vi "ValueChanged Callback.vi"(4 "onValueChanged":refnum<user-event>, 5 "Event Data":cluster{"sender":refnum<k24>, "e":refnum<k24>}, 6 "Control Ref":refnum<k24>, 7 "Event Common Data":T1) -> ()   [LabVIEW 2024, in "SourceGrid.lvlib" / "Custom Events.lvclass"]
uses:
  Custom Events.lvclass
  D:/git/Sourcegrid-LabVIEW/dll/SourceGrid.dll
  dll/SourceGrid.dll
  Cells/Cell Context/Cell Context.lvclass
  Custom Events.lvclass/Custom Events.ctl
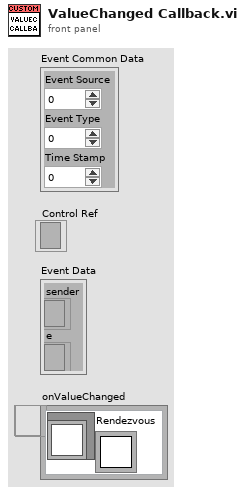
[diagram p1: front panel]
types:
  T1 = cluster{"Event Source":i32, "Event Type":u32, "Time Stamp":u32}
  T2 = typedef "Rendezvous RefNum" = refnum<k1>
  T3 = cluster{"Cell Context":refnum<class "Cell Context.lvclass">, "Rendezvous":T2}
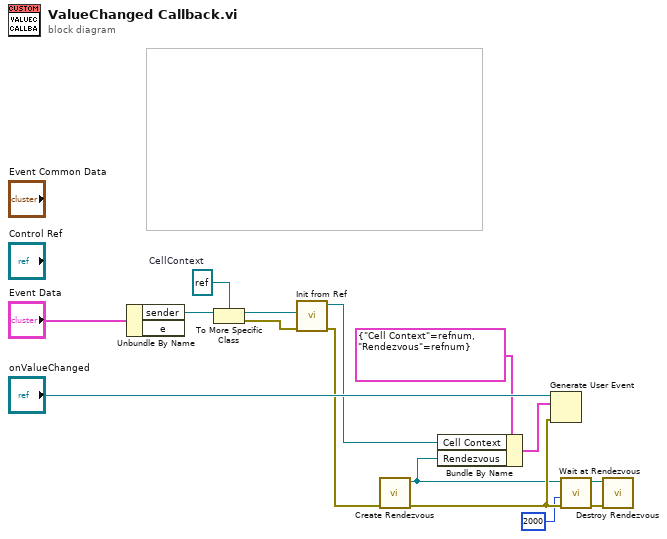
[diagram p0: block diagram]
diagram:
  w14 = refnum<k24> refnum  # CellContext
  n1 = Unbundle By Name("Event Data") -> ("sender"=w15:refnum<k24>)  [unwired: 1 out]
  n2 = To More Specific Class(target class=w14, reference=w15) -> (specific class reference=w10:refnum<k24>, error out=w13:errorcluster)  [unwired: 1 in]
  n3 = call "Init from Ref.vi"("error in"=w13, "CellContext .NET"=w10) -> ("error out"=w6:errorcluster, "Cell Context out"=w8:refnum<class "Cell Context.lvclass">)  [unwired: 8 in]
  n4 = call <vilib>:"Create Rendezvous.vi"("error in (no error)"=w6) -> ("error out"=w5:errorcluster, "rendezvous"=w1:T2)  [unwired: 4 in, 1 out]
  n5 = Bundle By Name(cluster=T3 {"Cell Context"=refnum, "Rendezvous"=refnum} ("onClick 2"), "Cell Context"=w8, "Rendezvous"=w1) -> (w7:T3)
  n6 = Generate User Event(user event="onValueChanged", event data cluster=w7, error in=w5) -> ()  [unwired: 1 in, 2 out]
  n7 = call <vilib>:"Wait at Rendezvous.vi"("error in (no error)"=w5, "ms timeout (-1)"=2000, "rendezvous"=w1) -> ("error out"=w3:errorcluster, "rendezvous out"=w4:T2)  [unwired: 2 in, 1 out]
  n8 = call <vilib>:"Destroy Rendezvous.vi"("error in (no error)"=w3, "rendezvous"=w4) -> ()  [unwired: 4 in, 2 out]
